vi "read_data_linear_y_single(SubVI).vi"(8 "error in (no error)":errorcluster) -> (0 "error out":errorcluster, 3 "Array":string[](array[string]))   [LabVIEW 2014]
uses:
  <vilib>/xml/Load XML String.vi
  <vilib>/xml/Close Reference(Node).vi
  <vilib>/addons/internet/NI_InternetTK_Core_VIs.lvlib
  <vilib>/xml/NI_XML.lvlib
  <resource>/objmgr/DOMUserDefRef.rc
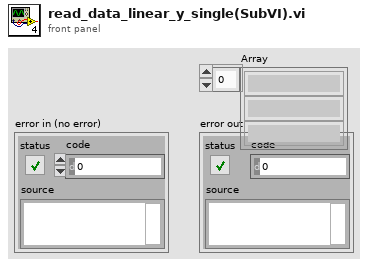
[diagram p1: front panel]
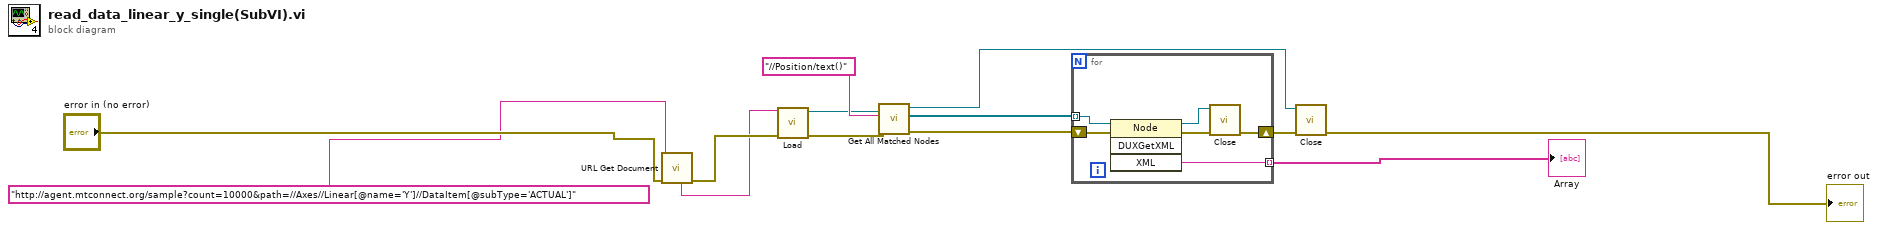
[diagram p0: block diagram]
diagram:
  n1 = call <vilib>:"URL Get Document.vi"("error in (no error)"="error in (no error)", "URL"="http://agent.mtconnect.org/sample?count=10000&path=//Axes//Linear[@name='Y']//DataItem[@subType='ACTUAL']") -> ("error out"=w11:errorcluster, "content"=w8:string)  [unwired: 5 in, 3 out]
  n2 = call-poly <vilib>:"Load.vi"("XML string"=w8, "error in (no error)"=w11) -> ("DOM document out"=w4:refnum<k20>, "error out"=w5:errorcluster)  [unwired: 11 in, 1 out]
  n3 = call <vilib>:"Get All Matched Nodes.vi"("error in (no error)"=w5, "XPath expression"="//Position/text()", "node in"=w4) -> ("error out"=w2:errorcluster, "node result array"=w1:refnum<k20>[], "node out"=w6:refnum<k20>)  [unwired: 6 out]
  n4 = for {
    tunnel: w1 -> [w15] mode=indexing
    shift-right: [w17] -> w3
    shift-left: w2 -> [w16]
    tunnel: [w14] -> w7 mode=indexing
    n5 = invoke on="Invoke Node" class="Node" method="DUXGetXML"(reference=w15, error in=w16) -> (reference out=w18:refnum<k20>, error out=w19:errorcluster, "XML"=w14:string)  [unwired: 2 in, 1 out]
    n6 = call-poly <vilib>:"Close.vi"("error in (no error)"=w19, "node"=w18) -> ("error out"=w17:errorcluster)  [unwired: 7 out]
  }
  "Array" <- w7
  n7 = call-poly <vilib>:"Close.vi"("error in (no error)"=w3, "node"=w6) -> ("error out"=→"error out":errorcluster)  [unwired: 7 out]
